vi "AcquireData.vi"(7 "Application Data":T1, 8 "error in (no error)":errorcluster, 11 "Acq Thread Data in":T2) -> (0 "error out":errorcluster, 3 "Acq Thread Data out":T2)   [LabVIEW 2019]
uses:
  Typedefs/Acquisition Thread/#cluster_AcqThreadData.ctl
  <vilib>/MagicBox/Device/Arduino/Arduino.lvclass
  <vilib>/MagicBox/Peripherals/POX/POX.lvclass
  Typedefs/Acquisition Thread/#enum_AcqThreadState.ctl
  Typedefs/#cluster_GUIRefs.ctl
  Typedefs/#cluster_ApplicationData.ctl
  Typedefs/Acquisition Thread/#cluster_AcqQueueData.ctl
  Typedefs/Acquisition Thread/#enum_AcquisitionTask.ctl
  Typedefs/Saving Thread/#cluster_SavingQueueData.ctl
  Typedefs/Saving Thread/#enum_SavingTask.ctl
  <vilib>/ActorFramework/Message Enqueuer/Message Enqueuer.lvclass
  <vilib>/MagicBox/Peripherals/POX/Read/Read Analog 1Smp 1Chl (Static, POX).vi
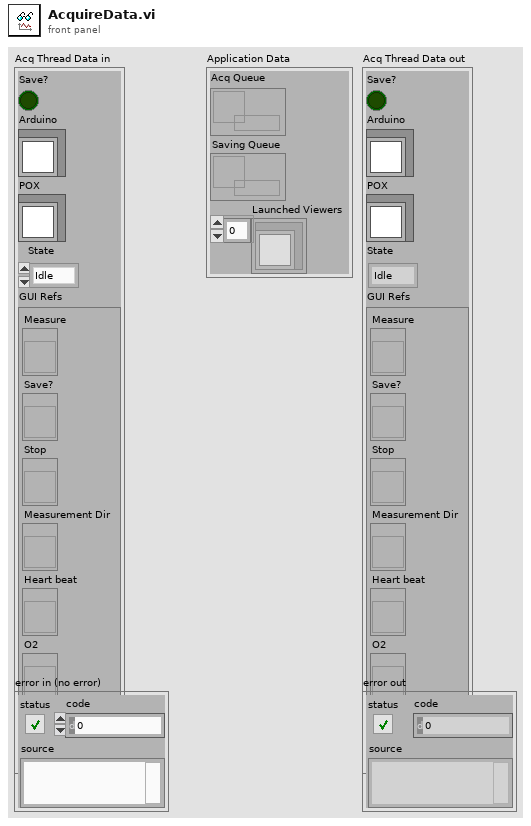
[diagram p1: front panel]
types:
  T1 = typedef "#cluster_ApplicationData.ctl" = cluster{"Acq Queue":refnum<queue>, "Saving Queue":refnum<queue>, "Launched Viewers":refnum<class "Message Enqueuer.lvclass">[]}
  T2 = typedef "#cluster_AcqThreadData.ctl" = cluster{"Save?":bool, "Arduino":refnum<class "Arduino.lvclass">, "POX":refnum<class "POX.lvclass">, "State":T3, "GUI Refs":T4}
  T3 = typedef "#enum_AcqThreadState.ctl" = enum16{"Idle", "Operate", "Error"}
  T4 = typedef "#cluster_GUIRefs.ctl" = cluster{"Measure":refnum<vi>, "Save?":refnum<vi>, "Stop":refnum<vi>, "Measurement Dir":refnum<vi>, "Heart beat":refnum<vi>, "O2":refnum<vi>, "POX Data History":refnum<vi>}
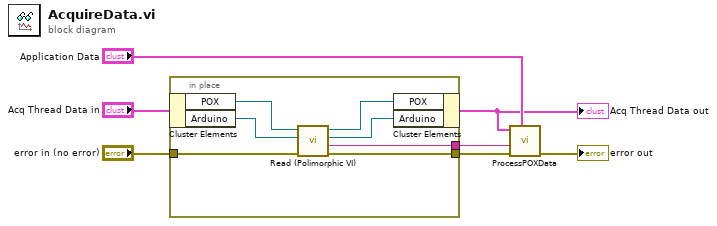
[diagram p0: block diagram]
diagram:
  n1 = in-place {
    in-place-border: "error in (no error)" -> [w14]
    in-place-border: [w13] -> w4
    in-place-border: [w8] -> w5
    n2 = in-place-cluster #1("Acq Thread Data in") -> ("POX"=w12:refnum<class "POX.lvclass">, "Arduino"=w11:refnum<class "Arduino.lvclass">)
    n3 = call-poly <vilib>:"Read (Polimorphic VI).vi"("error in (no error)"=w14, "Arduino in"=w11, "POX in"=w12) -> ("error out"=w13:errorcluster, "Read"=w8:string, "Arduino out"=w10:refnum<class "Arduino.lvclass">, "POX out"=w9:refnum<class "POX.lvclass">)  [unwired: 5 in]
    n4 = in-place-cluster #1("POX"=w9, "Arduino"=w10) -> (w1:T2)
  }
  "Acq Thread Data out" <- w1
  n5 = call "ProcessPOXData.vi"("Application Data"="Application Data", "error in (no error)"=w4, "POX Data"=w5, "Acq Thread Data in"=w1) -> ("error out"=→"error out":errorcluster)  [unwired: 7 in]
